vi "Tmplt init (SubVI).vi"(8 "error in":errorcluster, 10 "Template":u8[][](array[numeric]), 11 "Image Name":string="Tube") -> (0 "error out":errorcluster, 3 "Image Out":T1)   [LabVIEW 2013]
uses:
  <vilib>/vision/Image Controls.llb/IMAQ Image.ctl
  <vilib>/vision/NI_Vision_Development_Module.lvlib
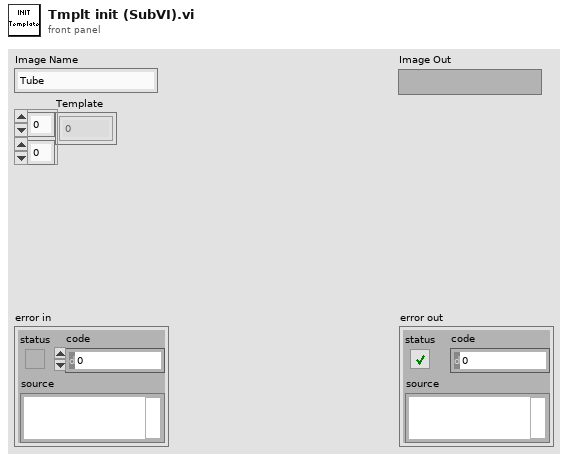
[diagram p1: front panel]
types:
  T1 = typedef "IMAQ Image.ctl" = refnum<image>
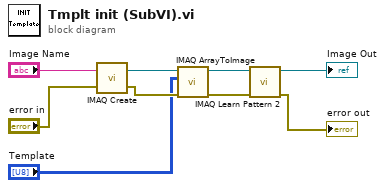
[diagram p0: block diagram]
diagram:
  n1 = call "IMAQ Create"("Image Name"="Image Name", "error in (no error)"="error in") -> ("New Image"=w8:T1, "error out"=w6:errorcluster)  [unwired: 3 in]
  n2 = call "IMAQ ArrayToImage"("error in (no error)"=w6, "Image Pixels (U8)"="Template", "Image"=w8) -> ("error out"=w5:errorcluster, "Image Out"=w7:T1)  [unwired: 7 in]
  n3 = call "IMAQ Learn Pattern 2"("error in (no error)"=w5, "Image"=w7) -> ("error out"=→"error out":errorcluster, "Template Image Out"=→"Image Out":T1)  [unwired: 8 in]
